vi "Launch Local Error Managers.vi"(8 "error in (no error)":errorcluster, 11 "Guardian in":refnum<class "Guardian.lvclass">) -> (0 "error out":errorcluster, 3 "Guardian out":refnum<class "Guardian.lvclass">)   [LabVIEW 2026, in "TALOS.lvlib" / "Guardian.lvlib" / "Guardian.lvclass"]
uses:
  Guardian.lvclass
  C:/LabVIEW Code/TALOS/talos/Ancestor/Ancestor/Ancestor.lvclass
  C:/LabVIEW Code/TALOS/builds/Actor Framework PPL/Actor Framework.lvlibp/1abvi3w/vi.lib/ActorFramework/Actor/Actor.lvclass
  Guardian Messages/Launch uService Msg/Launch uService Msg.lvclass/Launch uService Msg.ctl
  Ancestor/Ancestor/Read ID.vi
  builds/Actor Framework PPL/Actor Framework.lvlibp/1abvi3w/vi.lib/ActorFramework/Message Enqueuer/Enqueue.vi
  Guardian Messages/Launch uService Msg/Launch uService Msg.lvclass
  builds/Actor Framework PPL/Actor Framework.lvlibp/1abvi3w/vi.lib/ActorFramework/Actor/Actor.lvclass
  TALOS.lvlib
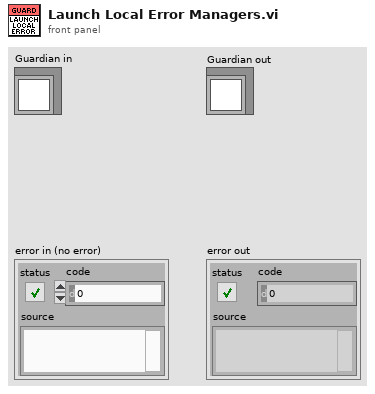
[diagram p1: front panel]
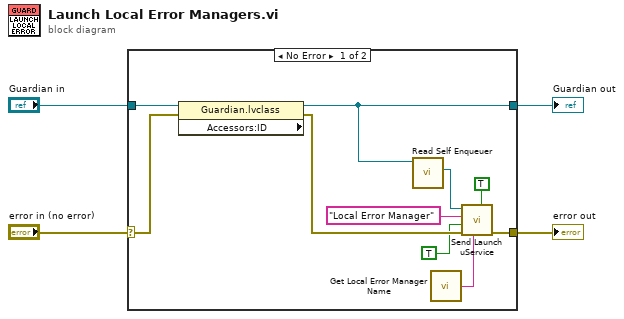
[diagram p0: block diagram]
diagram:
  n1 = case shown="No Error" "error in (no error)" {
    selector: "error in (no error)" -> [w8 w16]
    tunnel: "Guardian in" -> [w11 w15]
    tunnel: [w13 w16] -> w2
    tunnel: [w9 w15] -> w1
    frame No Error {
      n2 = property class="Guardian.lvclass" props=["Accessors:ID"](reference=w11, error in=w8) -> (reference out=w9:refnum<class "Guardian.lvclass">, error out=w10:errorcluster)  [unwired: 1 out]
      n3 = call "Read Self Enqueuer.vi"("Actor"=w9) -> ("Self Enqueuer"=w14:refnum<class "Message Enqueuer.lvclass">)  [unwired: 10 in]
      n4 = call "Get Local Error Manager Name.vi"() -> ("Error Manager ID"=w7:string)  [unwired: 1 in]
      n5 = call "Send Launch uService.vi"("Highlander?"=TRUE, "uService ID"=w7, "error in (no error)"=w10, "GUI?"=TRUE, "uService Class Name"="Local Error Manager", "Message Enqueuer"=w14) -> ("error out"=w13:errorcluster)  [unwired: 4 in, 1 out]
    }
    frame Error {
    }
  }
  "error out" <- w2
  "Guardian out" <- w1
